vi "Examen_01.vi"() -> ()   [LabVIEW 2017]
uses:
  <vilib>/Instr/_visa.llb/VISA Configure Serial Port (Instr).vi
panel:
  in  "stop":bool
  out "read buffer":string
  in  "VISA resource name":refnum<visa-resource-name>
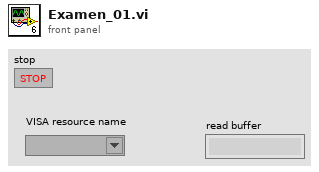
[diagram p1: front panel]
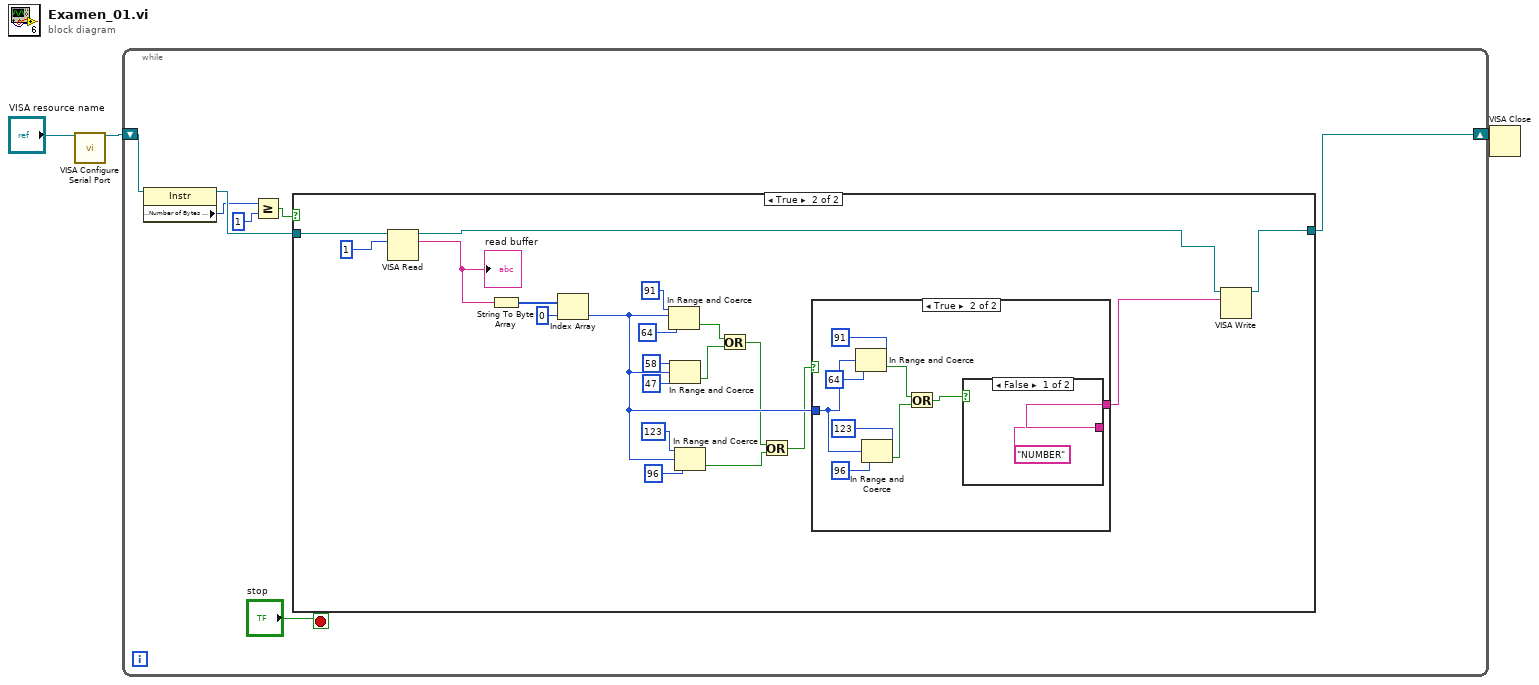
[diagram p0: block diagram]
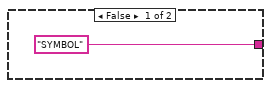
[diagram p3: hidden frame]
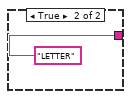
[diagram p4: hidden frame]
diagram:
  n1 = call-poly "VISA Configure Serial Port"("VISA resource name"="VISA resource name") -> ("VISA resource name out"=w2:refnum<visa-resource-name>)  [unwired: 13 in, 1 out]
  n2 = while {
    shift-right: [w4] -> w1
    shift-left: w2 -> [w9]
    stop <- "stop" stop-if-true
    n3 = property class="Instr"(reference=w9) -> (reference out=w8:refnum<visa-resource-name>, "Serial Settings:Number of Bytes at Serial Port"=w5:u32)  [unwired: 1 in, 1 out]
    n4 = Greater Or Equal?(x=w5, y=u32 1 ("x")) -> (x >= y?=w7:bool)
    n5 = case shown="True" w7 {
      tunnel: w8 -> [w11 w31]
      tunnel: [w11 w25] -> w4
      frame False {
      }
      frame True {
        n6 = VISA Read(VISA resource name=w31, byte count=u32 1) -> (VISA resource name out=w26:refnum<visa-resource-name>, read buffer=w29:string)  [unwired: 1 in, 2 out]
        "read buffer" <- w29
        n7 = String To Byte Array(string=w29) -> (unsigned byte array=w27:u8[])
        n8 = Index Array(array=w27, index=0) -> (element=w15:u8)
        n9 = In Range and Coerce(upper limit=u8 91, x=w15, lower limit=u8 64) -> (In Range?=w18:bool)  [unwired: 1 out]
        n10 = In Range and Coerce(upper limit=u8 58, x=w15, lower limit=u8 47) -> (In Range?=w19:bool)  [unwired: 1 out]
        n11 = In Range and Coerce(upper limit=u8 123, x=w15, lower limit=u8 96) -> (In Range?=w12:bool)  [unwired: 1 out]
        n12 = Or(x=w18, y=w19) -> (x .or. y?=w13:bool)
        n13 = Or(x=w13, y=w12) -> (x .or. y?=w14:bool)
        n14 = case shown="True" w14 {
          tunnel: ["SYMBOL" w39] -> w20
          tunnel: w15 -> [_ w34]
          frame False {
          }
          frame True {
            n15 = In Range and Coerce(upper limit=u8 91, x=w34, lower limit=u8 64) -> (In Range?=w37:bool)  [unwired: 1 out]
            n16 = In Range and Coerce(upper limit=u8 123, x=w34, lower limit=u8 96) -> (In Range?=w33:bool)  [unwired: 1 out]
            n17 = Or(x=w37, y=w33) -> (x .or. y?=w38:bool)
            n18 = case shown="False" w38 {
              tunnel: ["NUMBER" "LETTER"] -> w39
              frame False {
              }
              frame True {
              }
            }
          }
        }
        n19 = VISA Write(VISA resource name=w26, write buffer=w20) -> (VISA resource name out=w25:refnum<visa-resource-name>)  [unwired: 1 in, 2 out]
      }
    }
  }
  n20 = VISA Close(VISA resource name=w1) -> ()  [unwired: 1 in, 1 out]
